vi "PopulateMap.vi"() -> ()   [LabVIEW 2012]
doc: "This example shows how to use the mouse to draw circles in LabVIEW using the picture indicator and Property Nodes. This VI also shows how to change the color of the picture you draw and select whether it is an outlined circle or a filled circle.\n\nLabVIEW Version: 6.0.2\n\nINSTRUCTIONS:\n1. Run the VI.\n2. Select circle color by clicking the color box.\n3. To draw a filled circle, click the Fill Circle? button.\n4. Click anywhere inside the picture indicator.\n5. Drag the mouse.\n6. Release the mouse button.\n7. Repeat steps 4-6 as necessary.\n\nAuthor: \nNestor Sanchez\nApplications Engineer\nNational Instruments"
panel:
  out "Array":i32[][](array[numeric])
  in  "Path":path=path "C:/Users/wwarner/Documents/S4/RobotX/robot-x/Forebrain/Magical World/Mars1.png"
  in  "Use Blank":bool=TRUE
  in  "Radius":i16=10
  in  "Fill Circle?":bool=TRUE
  in  "stop":bool
  in  "Circle Color":u32(colorbox)=16724224
  out "600 by 600 Picture Map":picture
  # "Select Help»Show Context Help \nfor more information about using \nthis VI."
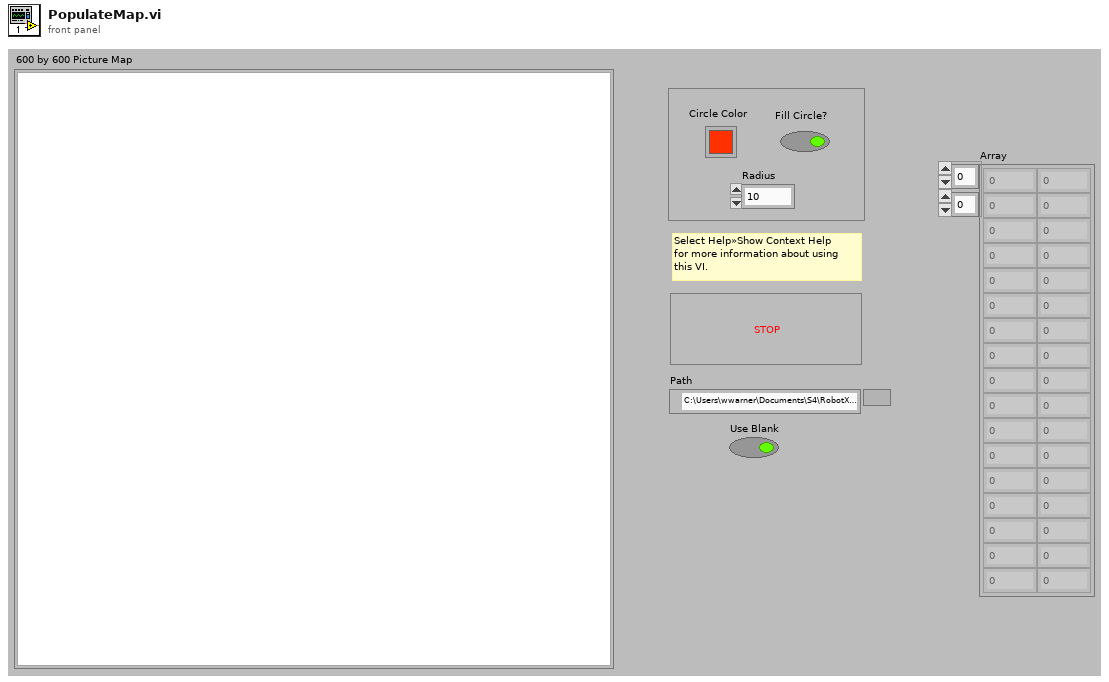
[diagram p1: front panel]
types:
  T1 = typedef "imagedata.ctl" = cluster{"image type":i32, "image depth":i32, "image":u8[], "mask":u8[], "colors":u32[], "Rectangle":cluster{"left":i16, "top":i16, "right":i16, "bottom":i16}}
  T2 = typedef "LVBoundsTypeDef.ctl" = cluster{"Width":u32, "Height":u32}
  T3 = typedef "LVMouseTypeDef.ctl" = cluster{"Mouse Position":cluster{"X":i32, "Y":i32}, "Mouse Modifiers":cluster{"Button Down":bool, "Shift Mod":bool, "Menu Mod":bool, "Option Mod":bool}}
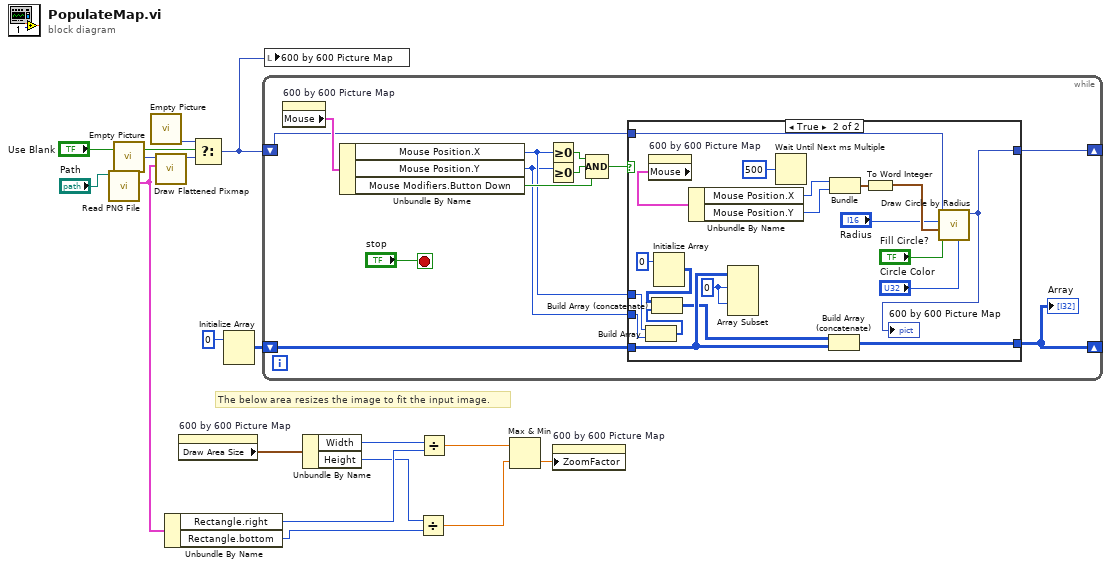
[diagram p0: block diagram]
diagram:
  # "The below area resizes the image to fit the input image."
  n1 = call <vilib>:"Read PNG File.vi"("path to PNG file"="Path") -> ("image data"=w11:T1)  [unwired: 8 in, 2 out]
  n2 = call "Empty Picture"() -> ("empty picture"=w14:picture)
  n3 = call "Empty Picture"() -> ("empty picture"=w12:picture)
  n4 = call <vilib>:"Draw Flattened Pixmap.vi"("image data"=w11, "picture"=w14) -> ("new picture"=w13:picture)  [unwired: 7 in]
  n5 = Unbundle By Name(w11) -> ("Rectangle.right"=w8:i16, "Rectangle.bottom"=w6:i16)
  n6 = property on="600 by 600 Picture Map" class="Pict"() -> ("Draw Area Size"=w10:T2)  [unwired: 2 in, 2 out]
  n7 = Select(t=w12, s="Use Blank", f=w13) -> (s? t:f=w17:picture)
  n8 = Initialize Array(0 ("element")) -> (w2:i32[][])  [unwired: 2 in]
  n9 = while {
    shift-right: [w23] -> _
    shift-left: w17 -> [w20]
    shift-right: [w18] -> _
    shift-left: w2 -> [w19]
    stop <- "stop" stop-if-true
    n10 = property on="600 by 600 Picture Map" class="Pict"() -> ("Mouse"=w29:T3)  [unwired: 2 in, 2 out]
    n11 = Unbundle By Name(w29) -> ("Mouse Position.X"=w22:i32, "Mouse Position.Y"=w21:i32, "Mouse Modifiers.Button Down"=w25:bool)
    n12 = Greater Or Equal To 0?(x=w22) -> (x >= 0?=w27:bool)
    n13 = Greater Or Equal To 0?(x=w21) -> (x >= 0?=w26:bool)
    n14 = Compound Arithmetic op=AND(w27, w26, w25) -> (w24:bool)
    n15 = case shown="True" w24 {
      tunnel: w22 -> [_ w36]
      tunnel: w21 -> [_ w37]
      tunnel: [w31 w51] -> w23
      tunnel: w20 -> [w31 w50]
      tunnel: w19 -> [w30 w34]
      tunnel: [w30 w33] -> w18
      frame False {
        # "When False do not do anything \nbut maintaining the picture \nalready draw."
      }
      frame True {
        w40 = 0 ("index")
        n16 = Build Array(w36, w37) -> (w35:i32[])
        n17 = property on="600 by 600 Picture Map" class="Pict"() -> ("Mouse"=w45:T3)  [unwired: 2 in, 2 out]
        n18 = Initialize Array(0 ("element")) -> (w38:i32[][])  [unwired: 2 in]
        n19 = Build Array (concatenate)(w38, w35) -> (w32:i32[][])
        n20 = Unbundle By Name(w45) -> ("Mouse Position.X"=w43:i32, "Mouse Position.Y"=w44:i32)
        n21 = Array Subset(array=w34, index (row)=w40, index (col)=w40) -> ()  [unwired: 2 in, 1 out]
        n22 = Wait Until Next ms Multiple(millisecond multiple=u32 500) -> ()  [unwired: 1 out]
        n23 = Build Array (concatenate)(w32, w34) -> (w33:i32[][])
        n24 = Bundle("X"=w43, "Y"=w44) -> (w49:cluster{"X":i32, "Y":i32})  [unwired: 1 in]
        n25 = To Word Integer(number=w49) -> (16bit integer=w46:cluster{"X":i16, "Y":i16})
        n26 = call <vilib>:"Draw Circle by Radius.vi"("color(black)"="Circle Color", "fill?(F)"="Fill Circle?", "pixel center"=w46, "radius"="Radius", "picture"=w50) -> ("new picture"=w51:picture)  [unwired: 6 in]
        "600 by 600 Picture Map" <- w51
      }
    }
    "Array" <- w18
  }
  n27 = local write "600 by 600 Picture Map"(w17) -> ()
  n28 = Unbundle By Name(w10) -> ("Width"=w9:u32, "Height"=w7:u32)
  n29 = Divide(x=w7, y=w6) -> (x/y=w4:dbl)
  n30 = Divide(x=w9, y=w8) -> (x/y=w5:dbl)
  n31 = Max & Min(x=w5, y=w4) -> (min(x,y)=w3:dbl)  [unwired: 1 out]
  n32 = property on="600 by 600 Picture Map" class="Pict"("ZoomFactor"=w3) -> ()  [unwired: 2 in, 2 out]
